vi "MCDC3006 Module.vi"(7 "Actions":T4(ring), 8 "Error In":errorcluster, 9 "Limits [In]":T2, 10 "Configuration [In]":T1, 11 "VISA resource name":refnum<visa-resource-name>="COM4") -> (0 "Error Out":errorcluster, 1 "Limits Out":T2, 2 "Configuration [Out]":T1, 4 "Status [Out]":T3, 5 "Active?":bool)   [LabVIEW 2018]
doc: "There are several actions that this VI can execute. \n\nOpen Session: Opens a VISA session at the VISA resource name\nClose Session: Closes the active VISA session\nSet/Get Configuration: Sets/Gets the Source Velocity, Mode and Target RPM\nEnable/Disable Motor: Enables or Disables the motor output on the controller\nGet Status: Gets the Instantaneous Motor Temperature, Velocity and Current draw\nSet/Get Limits: Sets/Gets the Peak and Constant Current Limits\nActive?: Reports current connection status of the controller? (read only)"
uses:
  General/Controls/Low Level Com Actions.ctl
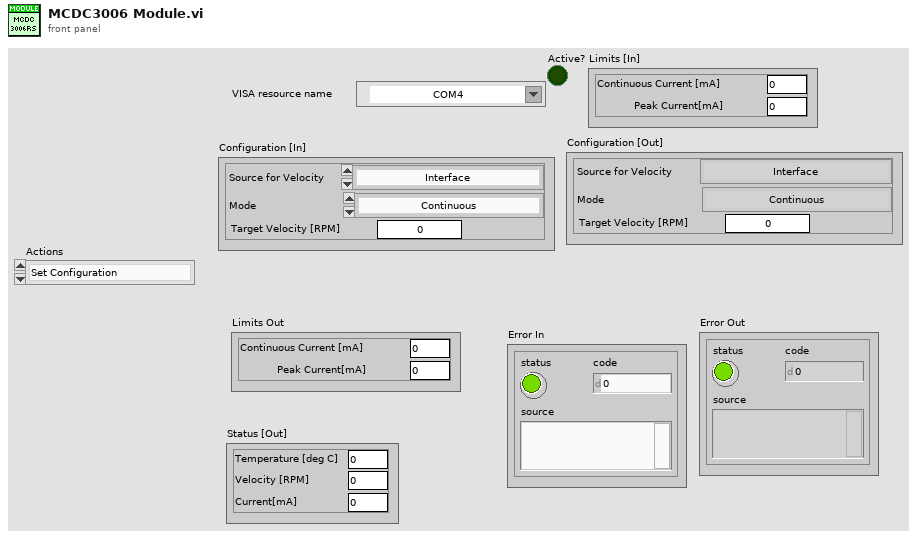
[diagram p1: front panel]
types:
  T1 = cluster{"Source for Velocity":enum16{"Interface", "Voltage (AI)", "PWM (AI)", "Current Target (AI)", "Current Target w/ Preset (AI)"}, "Mode":enum16{"Continuous", "Stepper Motor", "Analog Position Ctrl", "Encoder"}, "Target Velocity [RPM]":i16}
  T2 = cluster{"Continuous Current [mA]":dbl, "Peak Current[mA] ":dbl}
  T3 = cluster{"Temperature [deg C]":dbl, "Velocity [RPM]":dbl, "Current[mA] ":dbl}
  T4 = enum16{"Set Configuration", "Get Configuration", "Enable Motor", "Disable Motor", "Get Status", "Open Session", "Close Session", "Set Limits", "Get Limits"}
  T5 = typedef "Low Level Com Actions.ctl" = enum16{"Open Session", "Close Session", "Send Command", "Query Command"}
  T6 = enum16{"Interface", "Voltage (AI)", "PWM (AI)", "Current Target (AI)", "Current Target w/ Preset (AI)"}
  T7 = enum16{"Continuous", "Stepper Motor", "Analog Position Ctrl", "Encoder"}
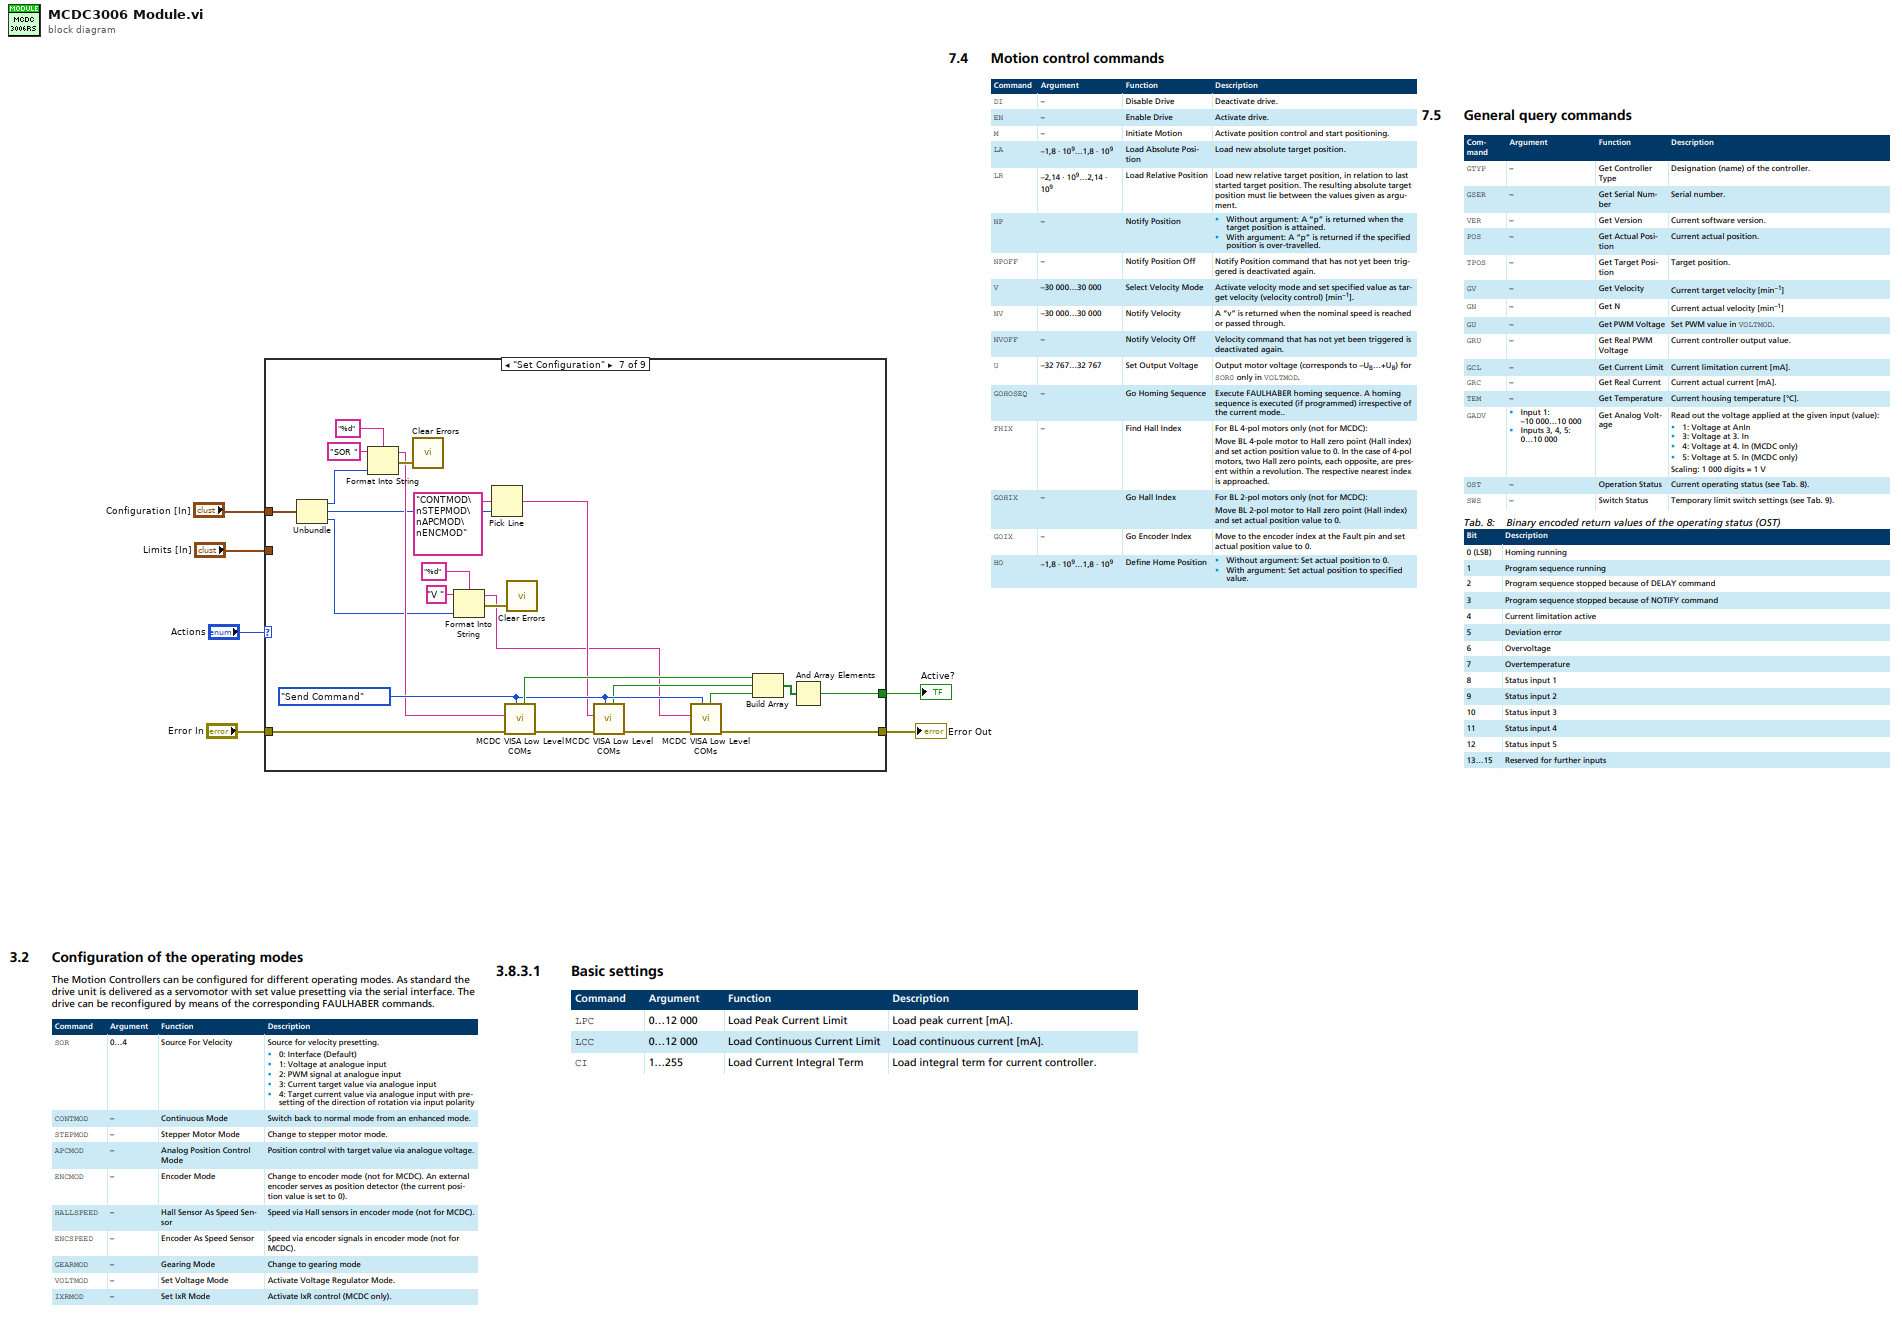
[diagram p0: block diagram]
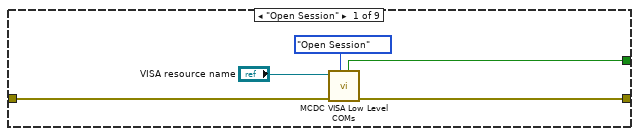
[diagram p2: hidden frame]
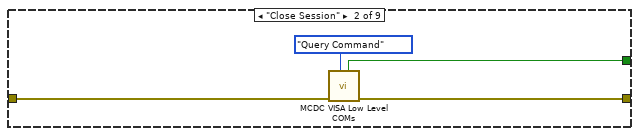
[diagram p3: hidden frame]
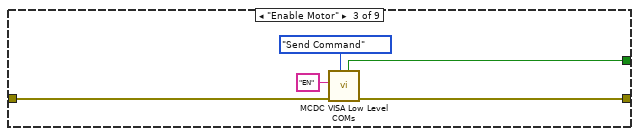
[diagram p4: hidden frame]
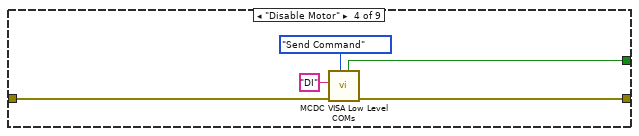
[diagram p5: hidden frame]
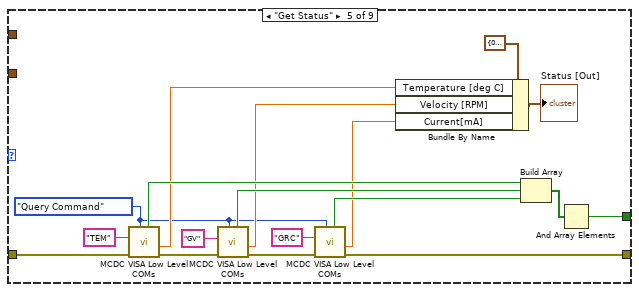
[diagram p6: hidden frame]
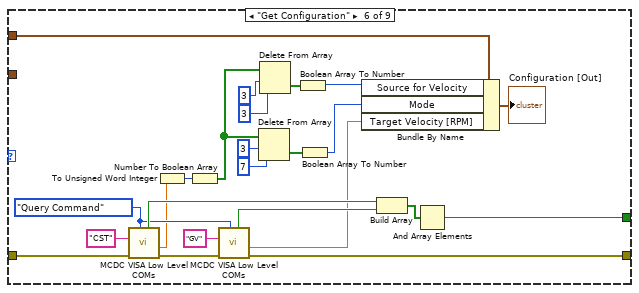
[diagram p7: hidden frame]
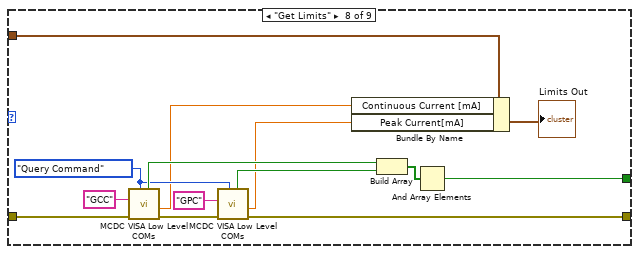
[diagram p8: hidden frame]
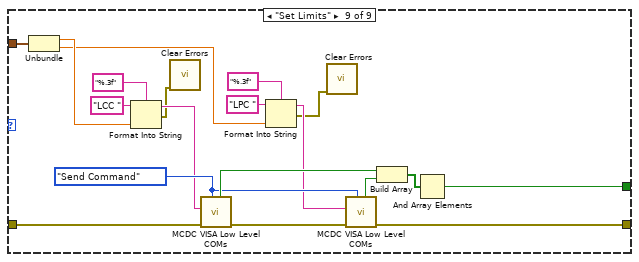
[diagram p9: hidden frame]
diagram:
  n1 = case shown="\"Set Configuration\"" "Actions" {
    tunnel: "Error In" -> [w10 w14 w19 w24 w43 w67 w91 w105 w124]
    tunnel: [w9 w13 w18 w23 w26 w62 w85 w93 w117] -> w5
    tunnel: [w7 w12 w17 w22 w41 w66 w89 w103 w122] -> w3
    tunnel: "Configuration [In]" -> [_ _ _ _ _ w56 w81 _ _]
    tunnel: "Limits [In]" -> [_ _ _ _ _ _ _ w92 w116]
    frame "Open Session" {
      n2 = call "MCDC VISA Low Level COMs.vi"("Action"=Low_Level_Com_Actions."Open Session", "error in (no error)"=w10, "VISA resource name"="VISA resource name") -> ("error out"=w9:errorcluster, "Active?"=w7:bool)  [unwired: 5 in, 2 out]
    }
    frame "Close Session" {
      n3 = call "MCDC VISA Low Level COMs.vi"("Action"=Low_Level_Com_Actions."Query Command", "error in (no error)"=w14) -> ("error out"=w13:errorcluster, "Active?"=w12:bool)  [unwired: 6 in, 2 out]
    }
    frame "Enable Motor" {
      n4 = call "MCDC VISA Low Level COMs.vi"("Action"=Low_Level_Com_Actions."Send Command", "error in (no error)"=w19, "Send Message"="EN") -> ("error out"=w18:errorcluster, "Active?"=w17:bool)  [unwired: 5 in, 2 out]
    }
    frame "Disable Motor" {
      n5 = call "MCDC VISA Low Level COMs.vi"("Action"=Low_Level_Com_Actions."Send Command", "error in (no error)"=w24, "Send Message"="DI") -> ("error out"=w23:errorcluster, "Active?"=w22:bool)  [unwired: 5 in, 2 out]
    }
    frame "Get Status" {
      w29 = Low_Level_Com_Actions."Query Command" ("Action")
      n6 = call "MCDC VISA Low Level COMs.vi"("Action"=w29, "error in (no error)"=w43, "Send Message"="TEM") -> ("error out"=w42:errorcluster, "Value"=w32:dbl, "Active?"=w39:bool)  [unwired: 5 in, 1 out]
      n7 = call "MCDC VISA Low Level COMs.vi"("Action"=w29, "error in (no error)"=w42, "Send Message"="GV") -> ("error out"=w37:errorcluster, "Value"=w31:dbl, "Active?"=w34:bool)  [unwired: 5 in, 1 out]
      n8 = call "MCDC VISA Low Level COMs.vi"("Action"=w29, "error in (no error)"=w37, "Send Message"="GRC") -> ("error out"=w26:errorcluster, "Value"=w30:dbl, "Active?"=w33:bool)  [unwired: 5 in, 1 out]
      n9 = Bundle By Name(cluster=T3 {"Temperature [deg C]"=0.0, "Velocity [RPM]"=0.0, "Current[mA] "=0.0} ("Status [In]"), "Temperature [deg C]"=w32, "Velocity [RPM]"=w31, "Current[mA]"=w30) -> (→"Status [Out]":T3)
      n10 = Build Array(w39, w34, w33) -> (w40:bool[])
      n11 = And Array Elements(Boolean array=w40) -> (logical AND=w41:bool)
    }
    frame "Get Configuration" {
      w60 = Low_Level_Com_Actions."Query Command" ("Action")
      n12 = call "MCDC VISA Low Level COMs.vi"("Action"=w60, "error in (no error)"=w67, "Send Message"="CST") -> ("error out"=w44:errorcluster, "Value"=w55:dbl, "Active?"=w64:bool)  [unwired: 5 in, 1 out]
      n13 = To Unsigned Word Integer(number=w55) -> (unsigned 16bit integer=w54:u16)
      n14 = Number To Boolean Array(number=w54) -> (Boolean array=w47:bool[])
      n15 = call "MCDC VISA Low Level COMs.vi"("Action"=w60, "error in (no error)"=w44, "Send Message"="GV") -> ("error out"=w62:errorcluster, "Value"=w58:dbl, "Active?"=w59:bool)  [unwired: 5 in, 1 out]
      n16 = Delete From Array(array=w47, length=3, index=7) -> (deleted portion=w51:bool[])  [unwired: 1 out]
      n17 = Delete From Array(array=w47, length=3, index=3) -> (deleted portion=w46:bool[])  [unwired: 1 out]
      n18 = Boolean Array To Number(Boolean array=w46) -> (number=w45:u32)
      n19 = Boolean Array To Number(Boolean array=w51) -> (number=w50:u32)
      n20 = Bundle By Name(cluster=w56, "Source for Velocity"=w45, "Mode"=w50, "Target Velocity [RPM]"=w58) -> (→"Configuration [Out]":T1)
      n21 = Build Array(w64, w59) -> (w65:bool[])
      n22 = And Array Elements(Boolean array=w65) -> (logical AND=w66:bool)
    }
    frame "Set Configuration" {
      w84 = Low_Level_Com_Actions."Send Command" ("Action")
      n23 = Unbundle(w81) -> ("Source for Velocity"=w78:T6, "Mode"=w75:T7, "Target Velocity [RPM]"=w69:i16)
      n24 = Format Into String(format string="%d", initial string="SOR " ("Send Message"), w78) -> (resulting string=w76:string, error out=w77:errorcluster)  [unwired: 1 in]
      n25 = call <vilib>:"Clear Errors.vi"("error in (no error)"=w77) -> ()  [unwired: 5 in, 2 out]
      n26 = Format Into String(format string="%d", initial string="V " ("Send Message"), w69) -> (resulting string=w68:string, error out=w72:errorcluster)  [unwired: 1 in]
      n27 = Pick Line(multi-line string="CONTMOD\nSTEPMOD\nAPCMOD\nENCMOD", line index=w75) -> (output string=w73:string)  [unwired: 1 in]
      n28 = call "MCDC VISA Low Level COMs.vi"("Action"=w84, "error in (no error)"=w91, "Send Message"=w76) -> ("error out"=w90:errorcluster, "Active?"=w87:bool)  [unwired: 5 in, 2 out]
      n29 = call <vilib>:"Clear Errors.vi"("error in (no error)"=w72) -> ()  [unwired: 5 in, 2 out]
      n30 = call "MCDC VISA Low Level COMs.vi"("Action"=w84, "error in (no error)"=w90, "Send Message"=w73) -> ("error out"=w86:errorcluster, "Active?"=w83:bool)  [unwired: 5 in, 2 out]
      n31 = call "MCDC VISA Low Level COMs.vi"("Action"=w84, "error in (no error)"=w86, "Send Message"=w68) -> ("error out"=w85:errorcluster, "Active?"=w82:bool)  [unwired: 5 in, 2 out]
      n32 = Build Array(w87, w83, w82) -> (w88:bool[])
      n33 = And Array Elements(Boolean array=w88) -> (logical AND=w89:bool)
    }
    frame "Get Limits" {
      w98 = Low_Level_Com_Actions."Query Command" ("Action")
      n34 = call "MCDC VISA Low Level COMs.vi"("Action"=w98, "error in (no error)"=w105, "Send Message"="GCC") -> ("error out"=w104:errorcluster, "Value"=w96:dbl, "Active?"=w101:bool)  [unwired: 5 in, 1 out]
      n35 = call "MCDC VISA Low Level COMs.vi"("Action"=w98, "error in (no error)"=w104, "Send Message"="GPC") -> ("error out"=w93:errorcluster, "Value"=w95:dbl, "Active?"=w97:bool)  [unwired: 5 in, 1 out]
      n36 = Bundle By Name(cluster=w92, "Continuous Current [mA]"=w96, "Peak Current[mA]"=w95) -> (→"Limits Out":T2)
      n37 = Build Array(w101, w97) -> (w102:bool[])
      n38 = And Array Elements(Boolean array=w102) -> (logical AND=w103:bool)
    }
    frame "Set Limits" {
      w119 = Low_Level_Com_Actions."Send Command" ("Action")
      n39 = Unbundle(w116) -> ("Continuous Current [mA]"=w114:dbl, "Peak Current[mA]"=w109:dbl)
      n40 = Format Into String(format string="%.3f", initial string="LCC " ("Send Message"), w114) -> (resulting string=w112:string, error out=w107:errorcluster)  [unwired: 1 in]
      n41 = call <vilib>:"Clear Errors.vi"("error in (no error)"=w107) -> ()  [unwired: 5 in, 2 out]
      n42 = call "MCDC VISA Low Level COMs.vi"("Action"=w119, "error in (no error)"=w124, "Send Message"=w112) -> ("error out"=w123:errorcluster, "Active?"=w120:bool)  [unwired: 5 in, 2 out]
      n43 = Format Into String(format string="%.3f", initial string="LPC " ("Send Message"), w109) -> (resulting string=w108:string, error out=w106:errorcluster)  [unwired: 1 in]
      n44 = call <vilib>:"Clear Errors.vi"("error in (no error)"=w106) -> ()  [unwired: 5 in, 2 out]
      n45 = call "MCDC VISA Low Level COMs.vi"("Action"=w119, "error in (no error)"=w123, "Send Message"=w108) -> ("error out"=w117:errorcluster, "Active?"=w118:bool)  [unwired: 5 in, 2 out]
      n46 = Build Array(w120, w118) -> (w121:bool[])
      n47 = And Array Elements(Boolean array=w121) -> (logical AND=w122:bool)
    }
  }
  "Error Out" <- w5
  "Active?" <- w3
